vi "launch pulsator vi.vi"(11 "messageHandler":T1 {"params"."controlChannels"."ballControl" items=["Module6/output0", "Module6/output1", "Module6/output2", "Module6/output3", "Not-Used"]; "params"."controlChannels"."butterflyControl" items=["Module6/output0", "Module6/output1", "Module6/output2", "Module6/output3", "Not-Used"]; "params"."controlChannels"."speedControl" items=["Module6/output0", "Module6/output1", "Module6/output2", "Module6/output3", "Not-Used"]}) -> ()   [LabVIEW 2018]
uses:
  type defs/message handler data.ctl
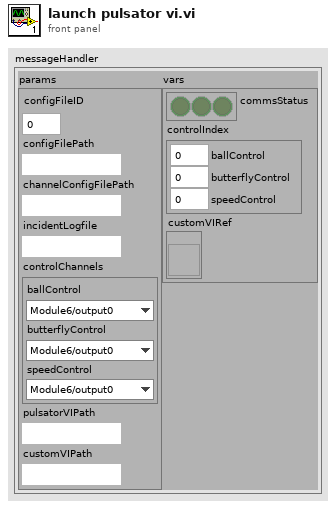
[diagram p1: front panel]
types:
  T1 = typedef "message handler data.ctl" = cluster{"params":cluster{"configFileID":u32, "configFilePath":path, "channelConfigFilePath":path, "incidentLogfile":path, "controlChannels":cluster{"ballControl":u16, "butterflyControl":u16, "speedControl":u16}, "pulsatorVIPath":path, "customVIPath":path}, "vars":cluster{"commsStatus":bool[], "controlIndex":cluster{"ballControl":u16, "butterflyControl":u16, "speedControl":u16}, "customVIRef":refnum<vi>}}
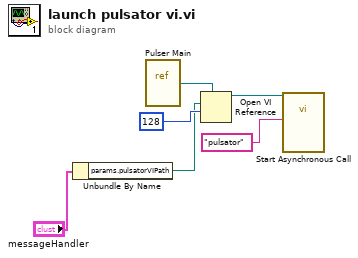
[diagram p0: block diagram]
diagram:
  n1 = Unbundle By Name("messageHandler") -> ("params.pulsatorVIPath"=w2:path)
  n2 = vi-ref "Pulser Main.vi"() -> (w4:refnum<vi>)
  n3 = Open VI Reference(type specifier VI Refnum (for type only)=w4, vi path=w2, options=128) -> (vi reference=w3:refnum<vi>)  [unwired: 3 in, 1 out]
  n4 = call-by-ref "Start Asynchronous Call"(reference=w3, "queue name"="pulsator") -> ()  [unwired: 12 in, 2 out]
